vi "NISE.Open Command.vi"   [LabVIEW 2016, in "SLSC Interface.lvclass"]
uses:
  SLSC Interface.lvclass
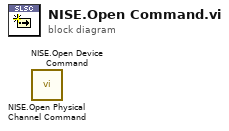
[diagram p0: block diagram]
diagram:
  n1 = call "NISE.Open Physical Channel Command.vi"() -> ()  [unwired: 13 in, 3 out]
  n2 = call "NISE.Open Device Command.vi"() -> ()  [unwired: 13 in, 3 out]
